vi "Pre Launch Init.vi"(11 "Project Builder in":refnum<class "Project Builder.lvclass">) -> (0 "error out":errorcluster, 3 "Project Builder out":refnum<class "Project Builder.lvclass">)   [LabVIEW 2014, in "Project Builder.lvclass"]
doc: "(<B>Filename</B>: Actor Framework.lvlib:Actor.lvclass:Pre Launch Init.vi)\n\nDefines behavior that occurs after the Launch Nested Actor method is invoked but before the actor's Actor Core method begins running.\n\nBy default, this method does nothing. A descendant class may override it to define behavior."
uses:
  Project Builder.lvclass
  Project Builder.lvclass/Project Builder.ctl
  <vilib>/ErrorRing/Error Ring.xnode
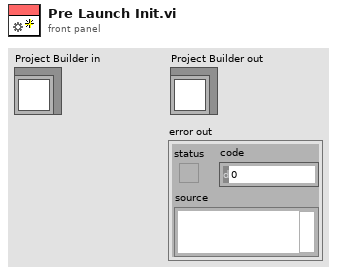
[diagram p1: front panel]
types:
  T1 = enum16{"open", "replace", "create", "open or create", "replace or create", "replace or create with confirmation"}
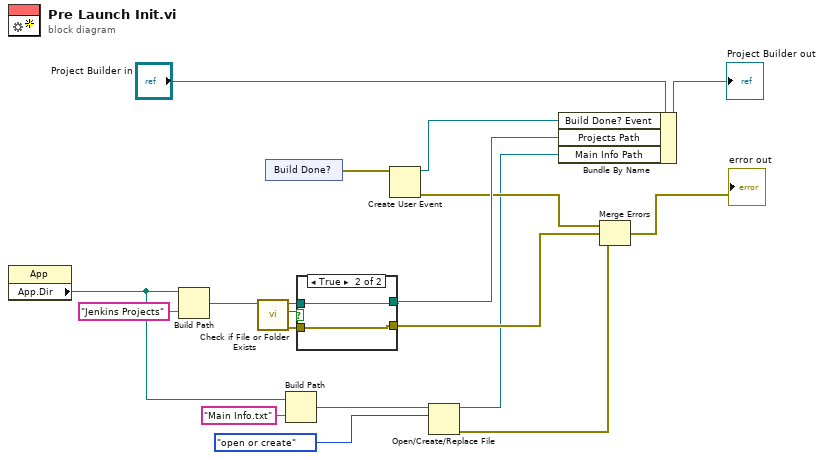
[diagram p0: block diagram]
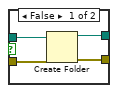
[diagram p2: hidden frame]
diagram:
  n1 = property class="App"() -> ("App.Dir"=w1:path)  [unwired: 2 in, 2 out]
  n2 = Build Path(base path=w1, name or relative path="Jenkins Projects") -> (appended path=w2:path)
  n3 = call <vilib>:"Check if File or Folder Exists.vi"("path"=w2) -> ("error out"=w13:errorcluster, "file or folder exists?"=w16:bool, "dup path"=w15:path)  [unwired: 8 in]
  n4 = xnode "Build Done?"() -> ("error out"=w3:errorcluster)
  n5 = Build Path(base path=w1, name or relative path="Main Info.txt") -> (appended path=w6:path)
  n6 = case shown="True" w16 {
    tunnel: w15 -> [w23 w25]
    tunnel: [w22 w25] -> w14
    tunnel: w13 -> [w21 w24]
    tunnel: [w20 w24] -> w12
    frame False {
      n7 = Create Folder(path (use dialog)=w23, error in=w21) -> (created path=w22:path, error out=w20:errorcluster)  [unwired: 1 in, 1 out]
    }
    frame True {
    }
  }
  n8 = Create User Event(user event datatype=w3) -> (user event=w18:refnum<user-event>, error out=w11:errorcluster)  [unwired: 1 in]
  n9 = Open/Create/Replace File(file path (use dialog)=w6, operation (0:open)=T1."open or create") -> (refnum out=w5:refnum<file>, error out=w4:errorcluster)  [unwired: 4 in, 1 out]
  n10 = Bundle By Name(cluster="Project Builder in", "Build Done? Event"=w18, "Projects Path"=w14, "Main Info Path"=w5) -> (→"Project Builder out":refnum<class "Project Builder.lvclass">)
  n11 = Merge Errors(w11, w12, w4) -> (→"error out":errorcluster)
